vi "Main.vi"() -> ()   [LabVIEW 2022 SP3]
doc: "This sample project is built upon the standard state machine template and shows how you could create an application that acquires, analyzes, and presents data. It includes functionality for presenting configuration dialogs, preserving settings between executions, loading and saving data, as well as exporting graph images and text files.\n\nIt is most appropriate for data that is acquired instantly as it does not allow for screen updates mid acquisition nor does it allow for continuous streaming to disk."
uses:
  controls/State.ctl
  controls/Data.ctl
  controls/UI References.ctl
  controls/Graph Data.ctl
  <vilib>/Utility/miscctls.llb/LVAnnotationListTypeDef.ctl
  <vilib>/Utility/miscctls.llb/LVCursorListTypeDef.ctl
  controls/User Specified Data.ctl
  controls/HW Configuration.ctl
  controls/Analysis Configuration.ctl
  controls/New Data Behavior.ctl
panel:
  in  "Settings":bool
  in  "Snapshot":bool
  in  "Analyze":bool
  in  "Clear":bool
  in  "Exit":bool
  in  "Acquire":bool
  in  "Export":bool
  in  "Save Data":bool
  in  "Load Data":bool
  out "Graph":waveform(dbl)[](graph)
  out "Status Bar":string
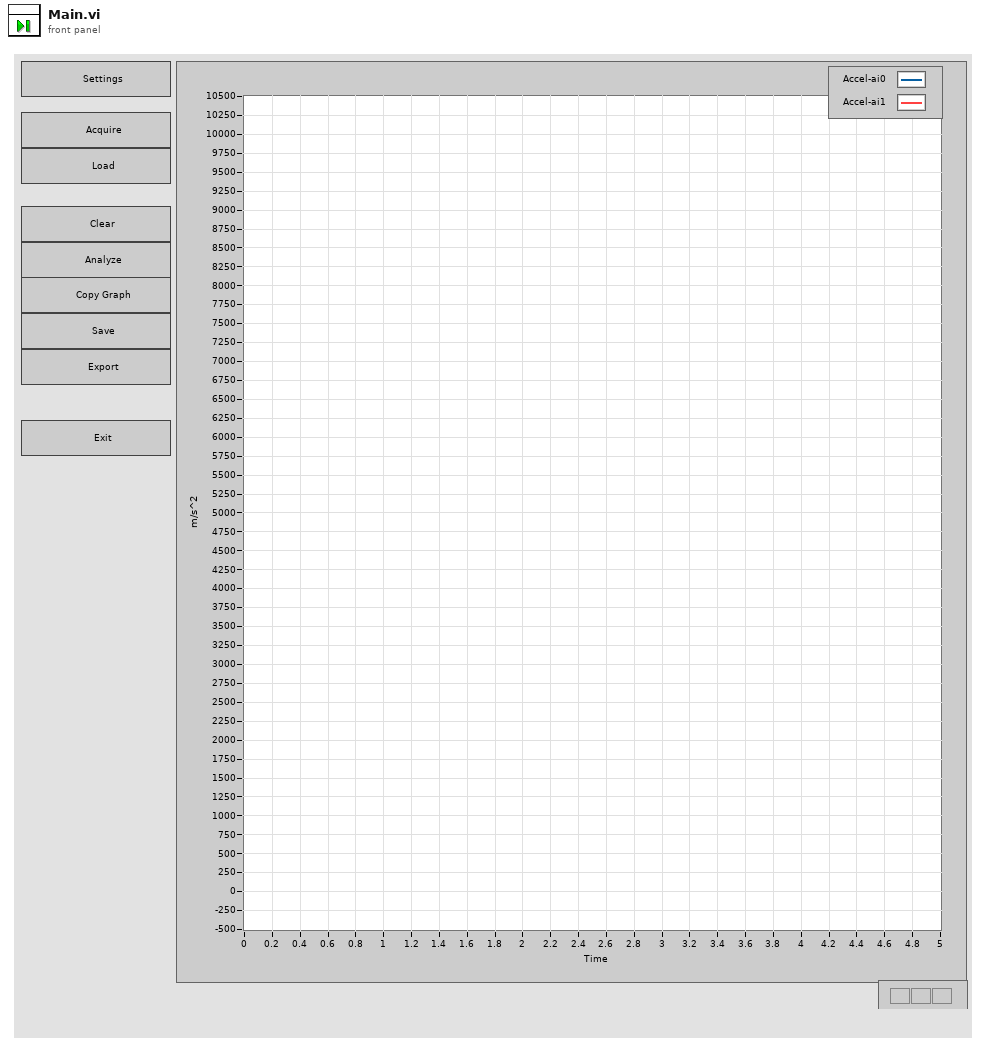
[diagram p1: front panel]
types:
  T1 = typedef "Data.ctl" = cluster{"UI References":T2, "Graph Data":T3, "User Specified":T6}
  T2 = typedef "UI References.ctl" = cluster{"Stop Ref":refnum<vi>, "Save Ref":refnum<vi>, "Open Ref":refnum<vi>, "Export Ref":refnum<vi>, "Acquire Ref":refnum<vi>, "Configure Ref":refnum<vi>, "Graph Ref":refnum<vi>, "Clear Ref":refnum<vi>, "Analyze Ref":refnum<vi>, "Status Ref":refnum<vi>, "Snapshot Ref":refnum<vi>}
  T3 = typedef "Graph Data.ctl" = cluster{"Data":waveform(dbl)[], "Annotation List":T4, "Cursor List":T5, "Analysis Data":waveform(dbl)[]}
  T4 = typedef "LVAnnotationListTypeDef.ctl" = cluster{"Name":string, "Color":u32, "Style":u8, "Point Style":u8, "Name Visible":bool, "Allow Drag":bool, "Annotation Mode":u32, "Plot":i32, "Index":i32, "Position":cluster{"X":dbl, "Y":dbl}, "X Scale":u32, "Y Scale":u32, "Show Arrow":bool, "Lock Name":bool, "Plot Area":i32, "Label Offset":cluster{"X":dbl, "Y":dbl}}[]
  T5 = typedef "LVCursorListTypeDef.ctl" = cluster{"Name":string, "Color":u32, "Style":u8, "Point Style":u8, "Name Visible":bool, "Allow Drag":bool, "Cursor Mode":u32, "Plot":i32, "Index":i32, "Position":cluster{"X":dbl, "Y":dbl}, "X Scale":u32, "Y Scale":u32, "Watch Plots":i32[], "Watch All Plots":bool, "Plot Area":i32, "Label Offset":cluster{"X":dbl, "Y":dbl}}[]
  T6 = typedef "User Specified Data.ctl" = cluster{"Hardware Configuration":T7, "Analysis Configuration":T8, "New Data Behavior":T9}
  T7 = typedef "HW Configuration.ctl" = cluster{"Accel-ai0":bool, "Maximum Input":dbl, "Minimum Input":dbl, "Sample Rate":dbl, "Number of Samples":i32, "Accel-ai1":bool}
  T8 = typedef "Analysis Configuration.ctl" = cluster{"Statistics":bool}
  T9 = typedef "New Data Behavior.ctl" = enum16{"Replace", "Overlay", "Append"}
  T10 = typedef "State.ctl" = enum16{"Initialize", "Wait for Event", "Update UI", "Configure", "Acquire", "Load Data", "Save Data", "Clear Data", "Export Data", "Analyze", "Copy Graph", "Exit"}
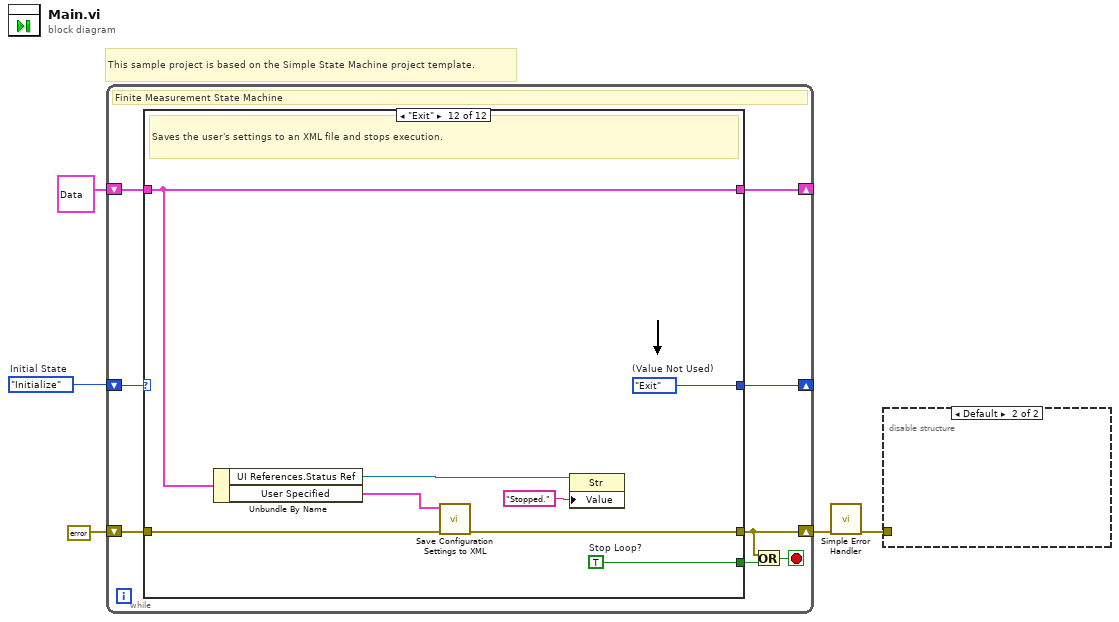
[diagram p0: block diagram]
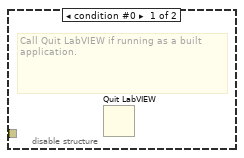
[diagram p2: hidden frame]
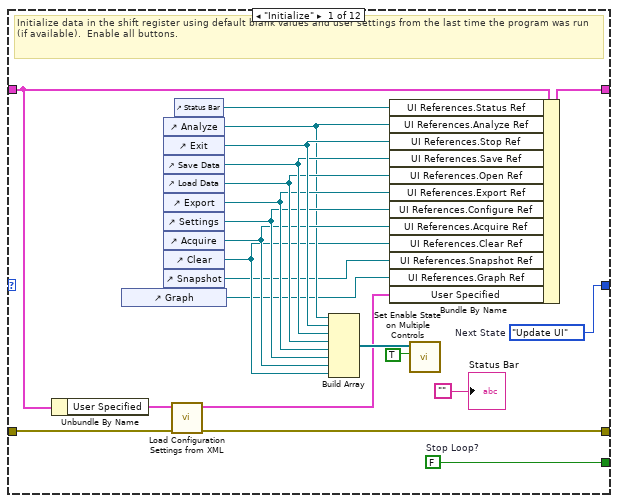
[diagram p3: hidden frame]
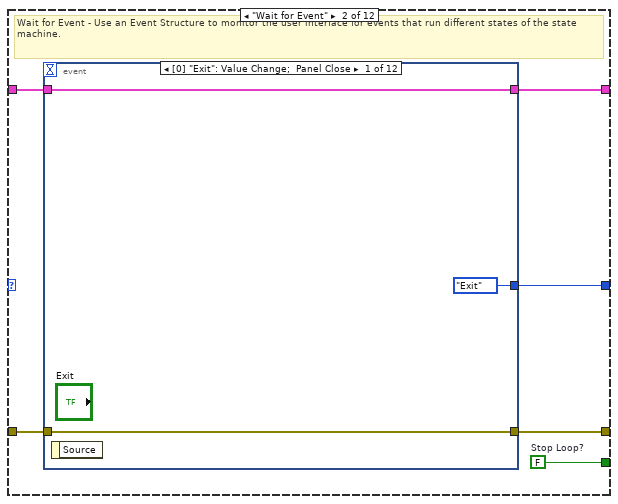
[diagram p4: hidden frame]
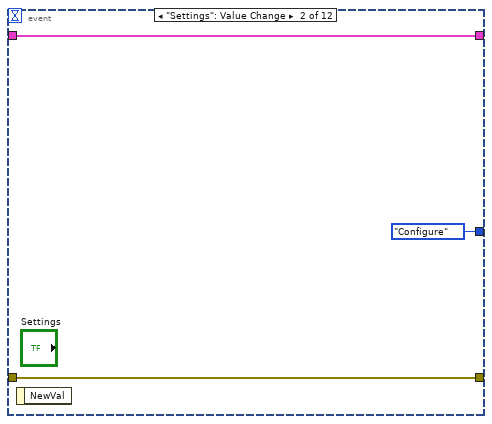
[diagram p5: hidden frame]
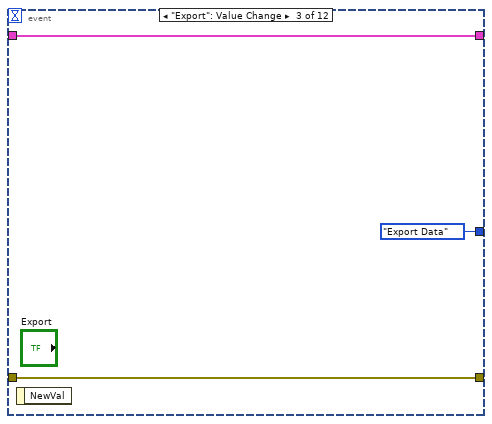
[diagram p6: hidden frame]
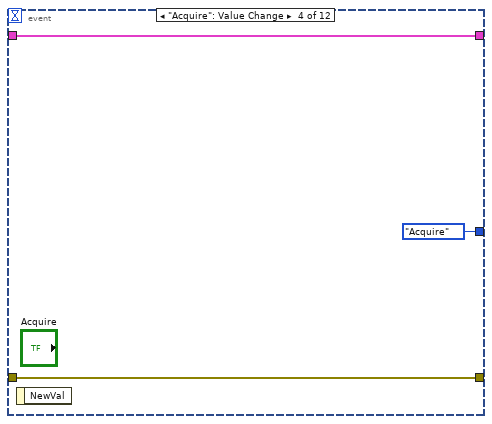
[diagram p7: hidden frame]
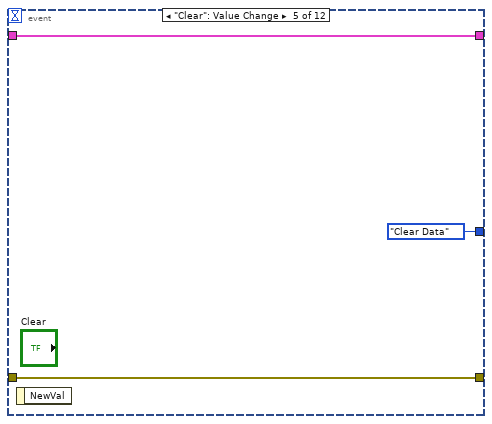
[diagram p8: hidden frame]
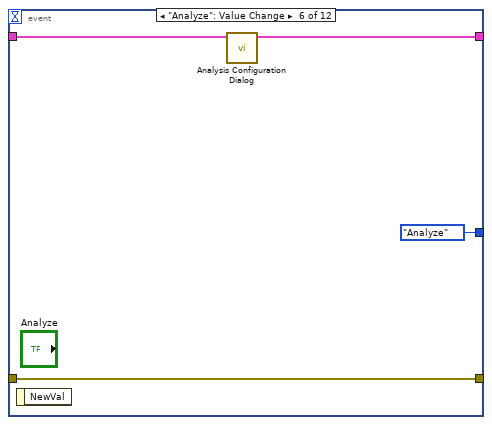
[diagram p9: hidden frame]
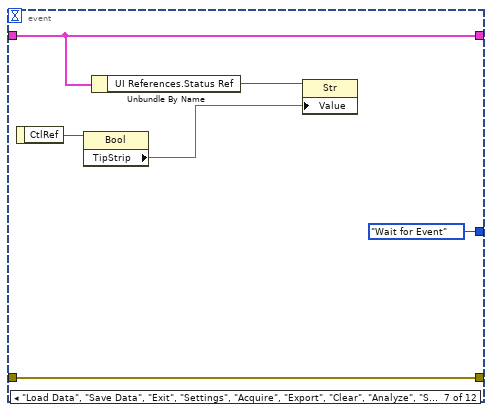
[diagram p10: hidden frame]
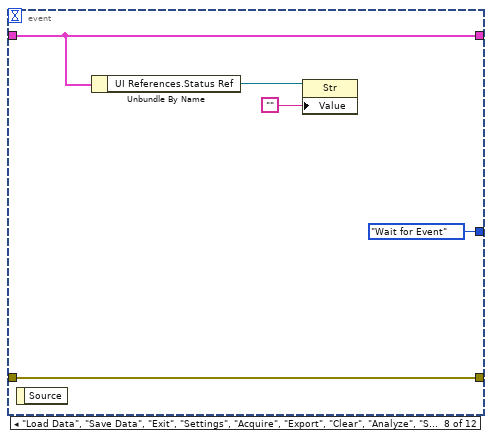
[diagram p11: hidden frame]
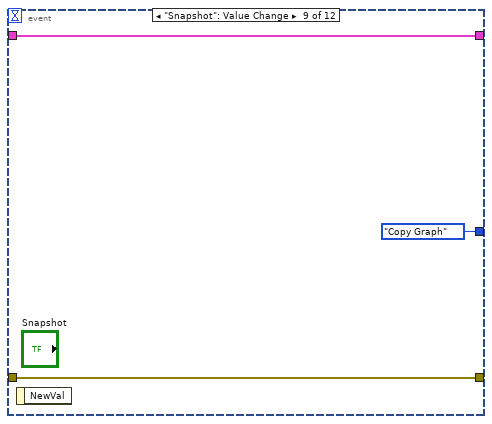
[diagram p12: hidden frame]
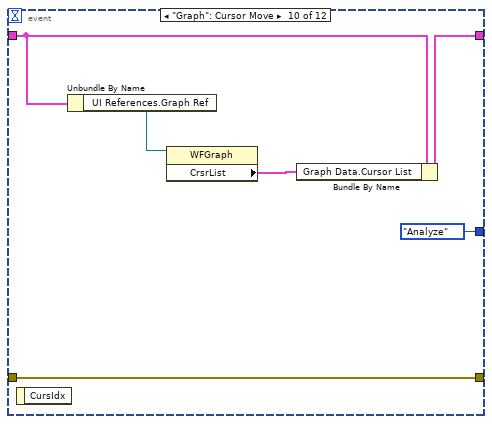
[diagram p13: hidden frame]
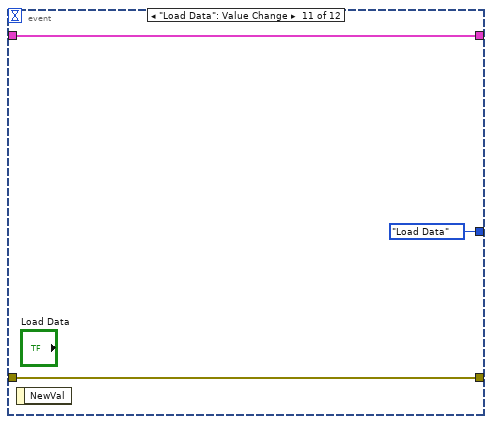
[diagram p14: hidden frame]
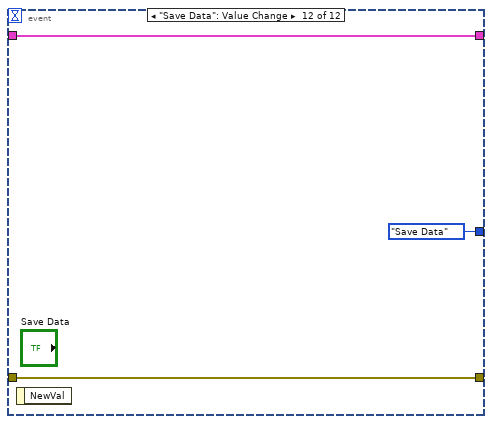
[diagram p15: hidden frame]
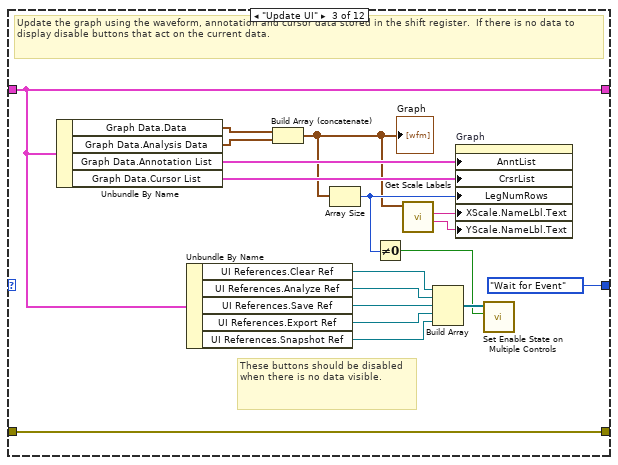
[diagram p16: hidden frame]
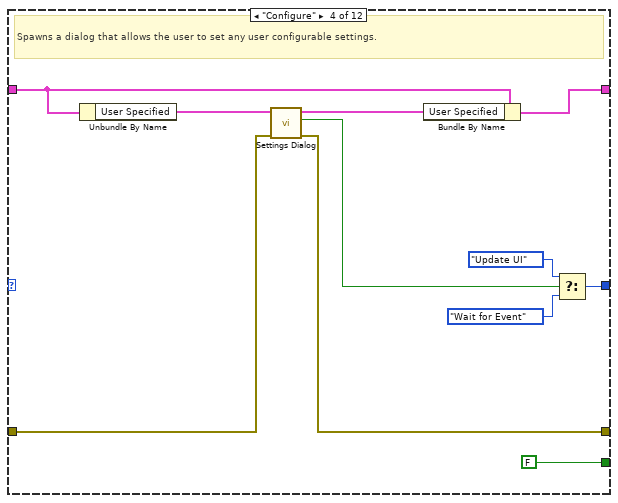
[diagram p17: hidden frame]
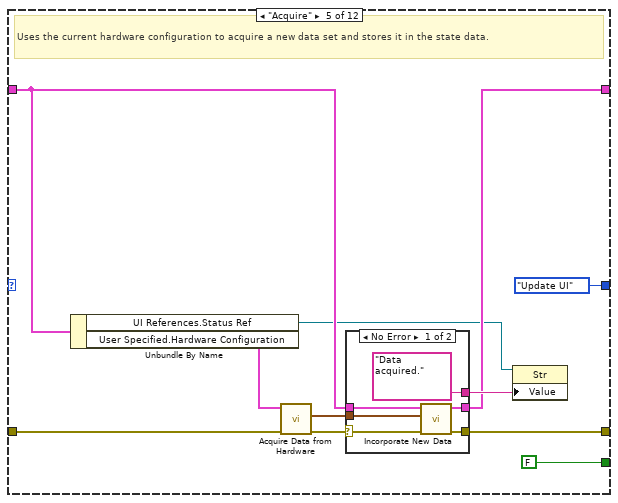
[diagram p18: hidden frame]
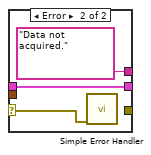
[diagram p19: hidden frame]
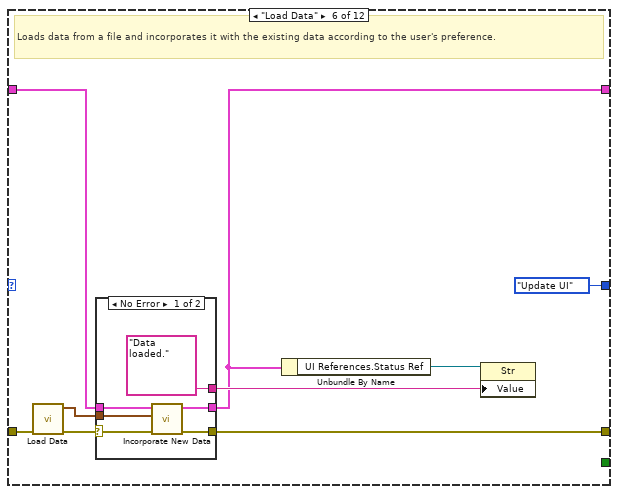
[diagram p20: hidden frame]
diagram:
  w5 = State."Initialize"  # Initial State
  # "This sample project is based on the Simple State Machine project template."
  n1 = while {
    shift-right: [w12] -> _
    shift-left: w5 -> [w13]
    shift-right: [w10] -> _
    shift-left: T1 {"UI References"={"Stop Ref"=refnum, "Save Ref"=refnum, "Open Ref"=refnum, "Export Ref"=refnum, "Acquire Ref"=refnum, "Configure Ref"=refnum, "Graph Ref"=refnum, "Clear Ref"=refnum, "Analyze Ref"=refnum, "Status Ref"=refnum, "Snapshot Ref"=refnum}, "Graph Data"={"Data"=[], "Annotation List"=[], "Cursor List"=[], "Analysis Data"=[]}, "User Specified"={"Hardware Configuration"={"Accel-ai0"=FALSE, "Maximum Input"=0.0, "Minimum Input"=0.0, "Sample Rate"=0.0, "Number of Samples"=0, "Accel-ai1"=FALSE}, "Analysis Configuration"={"Statistics"=FALSE}, "New Data Behavior"=enum."Replace"}} ("Data") -> [w11]
    shift-right: [w6] -> w2
    shift-left: errorcluster {"status"=FALSE, "code"=0, "source"=""} ("error constant") -> [w9]
    stop <- w7 stop-if-true
    # "Finite Measurement State Machine"
    n2 = case shown="\"Exit\"" w13 {
      tunnel: [w35 w41 State."Wait for Event" ("(Value Not Used)") w108 State."Update UI" ("Next State") State."Update UI" ("(Value Not Used)") State."Wait for Event" ("(Value Not Used)") State."Wait for Event" ("(Value Not Used)") State."Update UI" ("(Value Not Used)") State."Update UI" ("(Value Not Used)") State."Wait for Event" ("(Value Not Used)") w198] -> w12
      tunnel: [w34 w40 _ FALSE ("Stop Loop?") FALSE ("Stop Loop?") _ _ _ _ _ _ w197] -> w8
      tunnel: w11 -> [w25 w39 w101 w114 w121 w144 w157 w169 w180 w183 w189 w195]
      tunnel: [w33 w38 w101 w113 w120 w138 w157 w169 w179 w183 w189 w195] -> w10
      tunnel: w9 -> [w23 w37 w104 w112 w123 w143 w159 w172 w182 w185 w188 w192]
      tunnel: [w22 w36 w104 w111 w116 w142 w155 w166 w182 w185 w187 w191] -> w6
      frame "Initialize" {
        w34 = FALSE  # Stop Loop?
        w35 = State."Update UI"  # Next State
        # "Initialize data in the shift register using default blank values and user settings from the last time the program was run (if available).  Enable all buttons."
        n3 = Unbundle By Name(w25) -> ("User Specified"=w24:T6)
        n4 = control-ref of="Graph"() -> (w14:refnum<vi>)
        n5 = control-ref of="Analyze"() -> (w21:refnum<vi>)
        n6 = control-ref of="Exit"() -> (w32:refnum<vi>)
        n7 = control-ref of="Save Data"() -> (w31:refnum<vi>)
        n8 = control-ref of="Load Data"() -> (w30:refnum<vi>)
        n9 = control-ref of="Export"() -> (w29:refnum<vi>)
        n10 = control-ref of="Settings"() -> (w28:refnum<vi>)
        n11 = control-ref of="Acquire"() -> (w27:refnum<vi>)
        n12 = control-ref of="Clear"() -> (w19:refnum<vi>)
        n13 = control-ref of="Snapshot"() -> (w15:refnum<vi>)
        n14 = call "Load Configuration Settings from XML.vi"("error in (no error)"=w23, "User Configuration in"=w24) -> ("error out"=w22:errorcluster, "User Configuration out"=w17:T6)  [unwired: 8 in]
        n15 = control-ref of="Status Bar"() -> (w20:refnum<vi>)
        n16 = Build Array(w21, w32, w31, w30, w29, w28, w27, w19) -> (w26:refnum<vi>[])
        n17 = Bundle By Name(cluster=w25, "UI References.Status Ref"=w20, "UI References.Analyze Ref"=w21, "UI References.Stop Ref"=w32, "UI References.Save Ref"=w31, "UI References.Open Ref"=w30, "UI References.Export Ref"=w29, "UI References.Configure Ref"=w28, "UI References.Acquire Ref"=w27, "UI References.Clear Ref"=w19, "UI References.Snapshot Ref"=w15, "UI References.Graph Ref"=w14, "User Specified"=w17) -> (w33:T1)
        n18 = call "Set Enable State on Multiple Controls.vi"("Enable?"=TRUE, "Controls"=w26) -> ()  [unwired: 10 in]
        "Status Bar" <- "" ("Status Bar")
      }
      frame "Wait for Event" {
        w40 = FALSE  # Stop Loop?
        # "Wait for Event - Use an Event Structure to monitor the user interface for events that run different states of the state machine."
        n19 = event shown="[0] \"Exit\": Value Change;  Panel Close" {
          selector: _ -> [_ _ _ _ _ _ _ _ _ _ _ _]
          dyn-events: _ -> [_ _ _ _ _ _ _ _ _ _ _ _]
          timeout: _ -> [_ _ _ _ _ _ _ _ _ _ _ _]
          tunnel: [State."Exit" ("Next State") State."Configure" ("Next State") State."Export Data" ("Next State") State."Acquire" ("Next State") State."Clear Data" ("Next State") State."Analyze" ("Next State") State."Wait for Event" ("Next State") State."Wait for Event" ("Next State") State."Copy Graph" ("Next State") State."Analyze" ("Next State") State."Load Data" ("Next State") State."Save Data" ("Next State")] -> w41
          tunnel: w39 -> [w43 w47 w50 w53 w56 w58 w64 w70 w74 w75 w82 w85]
          tunnel: [w43 w47 w50 w53 w56 w57 w64 w70 w74 w78 w82 w85] -> w38
          tunnel: w37 -> [w42 w46 w49 w52 w55 w60 w66 w71 w73 w80 w81 w84]
          tunnel: [w42 w46 w49 w52 w55 w60 w66 w71 w73 w80 w81 w84] -> w36
          event "Exit": Value Change; Panel Close {
            n20 = event-data() -> ()  [unwired: 1 in, 1 out]
          }
          event "Settings": Value Change {
            n21 = event-data() -> ()  [unwired: 1 in, 1 out]
          }
          event "Export": Value Change {
            n22 = event-data() -> ()  [unwired: 1 in, 1 out]
          }
          event "Acquire": Value Change {
            n23 = event-data() -> ()  [unwired: 1 in, 1 out]
          }
          event "Clear": Value Change {
            n24 = event-data() -> ()  [unwired: 1 in, 1 out]
          }
          event "Analyze": Value Change {
            n25 = event-data() -> ()  [unwired: 1 in, 1 out]
            n26 = call "Analysis Configuration Dialog.vi"("Data in"=w58) -> ("Data out"=w57:T1)  [unwired: 10 in]
          }
          event "Load Data", "Save Data", "Exit", "Settings", "Acquire", "Export", "Clear", "Analyze", "Snapshot": Mouse Enter {
            n27 = event-data() -> ("CtlRef"=w65:refnum<vi>)  [unwired: 1 in]
            n28 = property class="Bool"(reference=w65) -> ("TipStrip"=w62:string)  [unwired: 1 in, 2 out]
            n29 = Unbundle By Name(w64) -> ("UI References.Status Ref"=w63:refnum<vi>)
            n30 = property class="Str"(reference=w63, "Value"=w62) -> ()  [unwired: 1 in, 2 out]
          }
          event "Load Data", "Save Data", "Exit", "Settings", "Acquire", "Export", "Clear", "Analyze", "Snapshot": Mouse Leave {
            n31 = event-data() -> ()  [unwired: 1 in, 1 out]
            n32 = Unbundle By Name(w70) -> ("UI References.Status Ref"=w69:refnum<vi>)
            n33 = property class="Str"(reference=w69, "Value"="") -> ()  [unwired: 1 in, 2 out]
          }
          event "Snapshot": Value Change {
            n34 = event-data() -> ()  [unwired: 1 in, 1 out]
          }
          event "Graph": Cursor Move {
            n35 = event-data() -> ()  [unwired: 1 in, 1 out]
            n36 = Unbundle By Name(w75) -> ("UI References.Graph Ref"=w77:refnum<vi>)
            n37 = property class="WFGraph"(reference=w77) -> ("CrsrList"=w76:T5)  [unwired: 1 in, 2 out]
            n38 = Bundle By Name(cluster=w75, "Graph Data.Cursor List"=w76) -> (w78:T1)
          }
          event "Load Data": Value Change {
            n39 = event-data() -> ()  [unwired: 1 in, 1 out]
          }
          event "Save Data": Value Change {
            n40 = event-data() -> ()  [unwired: 1 in, 1 out]
          }
        }
      }
      frame "Update UI" {
        # "These buttons should be disabled when there is no data visible."
        # "Update the graph using the waveform, annotation and cursor data stored in the shift register.  If there is no data to display disable buttons that act on the current data."
        n41 = Unbundle By Name(w101) -> ("Graph Data.Data"=w97:waveform(dbl)[], "Graph Data.Analysis Data"=w87:waveform(dbl)[], "Graph Data.Annotation List"=w102:T4, "Graph Data.Cursor List"=w98:T5)
        n42 = Unbundle By Name(w101) -> ("UI References.Clear Ref"=w93:refnum<vi>, "UI References.Analyze Ref"=w92:refnum<vi>, "UI References.Save Ref"=w100:refnum<vi>, "UI References.Export Ref"=w90:refnum<vi>, "UI References.Snapshot Ref"=w91:refnum<vi>)
        n43 = Build Array (concatenate)(w97, w87) -> (w95:waveform(dbl)[])
        "Graph" <- w95
        n44 = Array Size(array=w95) -> (size(s)=w96:i32)
        n45 = Not Equal To 0?(x=w96) -> (x != 0?=w94:bool)
        n46 = call "Get Scale Labels.vi"("Array of Waveforms"=w95) -> ("Y Scale Label Text"=w88:string, "X Scale Label Text"=w89:string)  [unwired: 9 in]
        n47 = Build Array(w93, w92, w100, w90, w91) -> (w99:refnum<vi>[])
        n48 = property on="Graph" class="WFGraph (strict)"("AnntList"=w102, "CrsrList"=w98, "LegNumRows"=w96, "XScale.NameLbl.Text"=w89, "YScale.NameLbl.Text"=w88) -> ()  [unwired: 2 in, 2 out]
        n49 = call "Set Enable State on Multiple Controls.vi"("Enable?"=w94, "Controls"=w99) -> ()  [unwired: 10 in]
      }
      frame "Configure" {
        # "Spawns a dialog that allows the user to set any user configurable settings."
        n50 = Unbundle By Name(w114) -> ("User Specified"=w106:T6)
        n51 = call "Settings Dialog.vi"("error in (no error)"=w112, "Configuration in"=w106) -> ("error out"=w111:errorcluster, "UI Refresh Needed?"=w110:bool, "Configuration out"=w105:T6)  [unwired: 7 in]
        n52 = Bundle By Name(cluster=w114, "User Specified"=w105) -> (w113:T1)
        n53 = Select(t=State."Update UI" ("Next State if true"), s=w110, f=State."Wait for Event" ("Next State if false")) -> (s? t:f=w108:T10)
      }
      frame "Acquire" {
        # "Uses the current hardware configuration to acquire a new data set and stores it in the state data."
        n54 = Unbundle By Name(w121) -> ("UI References.Status Ref"=w117:refnum<vi>, "User Specified.Hardware Configuration"=w124:T7)
        n55 = call "Acquire Data from Hardware.vi"("error in (no error)"=w123, "Hardware Configuration"=w124) -> ("error out"=w118:errorcluster, "Graph Data"=w119:waveform(dbl)[])  [unwired: 7 in]
        n56 = case shown="No Error" w118 {
          selector: w118 -> [w129 w134]
          tunnel: w121 -> [w128 w135]
          tunnel: [w132 w135] -> w120
          tunnel: [w131 _] -> w116
          tunnel: w119 -> [w130 _]
          tunnel: ["Data acquired." ("Data acquired") "Data not acquired." ("Data not acquired")] -> w122
          frame No Error {
            n57 = call "Incorporate New Data.vi"("error in (no error)"=w129, "New Graph Data"=w130, "Data in"=w128) -> ("error out"=w131:errorcluster, "Data out"=w132:T1)  [unwired: 7 in]
          }
          frame Error {
            n58 = call <vilib>:"Simple Error Handler.vi"("error in (no error)"=w134) -> ()  [unwired: 4 in, 5 out]
          }
        }
        n59 = property class="Str"(reference=w117, "Value"=w122) -> ()  [unwired: 1 in, 2 out]
      }
      frame "Load Data" {
        # "Loads data from a file and incorporates it with the existing data according to the user's preference."
        n60 = call "Load Data.vi"("error in (no error)"=w143) -> ("error out"=w140:errorcluster, "New Graph Data"=w137:waveform(dbl)[])  [unwired: 9 in]
        n61 = case shown="No Error" w140 {
          selector: w140 -> [w147 w152]
          tunnel: w144 -> [w146 w153]
          tunnel: [w150 w153] -> w138
          tunnel: [w149 _] -> w142
          tunnel: w137 -> [w148 _]
          tunnel: ["Data loaded." ("Data loaded") "Data not loaded." ("Data not loaded")] -> w139
          frame No Error {
            n62 = call "Incorporate New Data.vi"("error in (no error)"=w147, "New Graph Data"=w148, "Data in"=w146) -> ("error out"=w149:errorcluster, "Data out"=w150:T1)  [unwired: 7 in]
          }
          frame Error {
            n63 = call <vilib>:"Simple Error Handler.vi"("error in (no error)"=w152) -> ()  [unwired: 4 in, 5 out]
          }
        }
        n64 = Unbundle By Name(w138) -> ("UI References.Status Ref"=w136:refnum<vi>)
        n65 = property class="Str"(reference=w136, "Value"=w139) -> ()  [unwired: 1 in, 2 out]
      }
      frame "Save Data" {
        # "Saves the existing measurement data to a file."
        n66 = Unbundle By Name(w157) -> ("UI References.Status Ref"=w156:refnum<vi>, "Graph Data.Data"=w160:waveform(dbl)[])
        n67 = call "Save Data.vi"("error in (no error)"=w159, "Data"=w160) -> ("error out"=w158:errorcluster)  [unwired: 9 in]
        n68 = case shown="No Error" w158 {
          selector: w158 -> [w162 w165]
          tunnel: ["Data saved." ("Data saved") "Data not saved." ("Data not saved")] -> w154
          tunnel: [w162 _] -> w155
          frame No Error {
          }
          frame Error {
            n69 = call <vilib>:"Simple Error Handler.vi"("error in (no error)"=w165) -> ()  [unwired: 4 in, 5 out]
          }
        }
        n70 = property class="Str"(reference=w156, "Value"=w154) -> ()  [unwired: 1 in, 2 out]
      }
      frame "Export Data" {
        # "Exports the currently loaded measurement and analysis data to a text file that can be imported into a spreadsheet or other application."
        n71 = Unbundle By Name(w169) -> ("UI References.Status Ref"=w167:refnum<vi>, "Graph Data"=w168:T3)
        n72 = call "Export Data.vi"("error in (no error)"=w172, "Graph Data"=w168) -> ("error out"=w170:errorcluster)  [unwired: 9 in]
        n73 = case shown="No Error" w170 {
          selector: w170 -> [w174 w177]
          tunnel: ["Data exported." ("Data exported") "Data not exported." ("Data not exported")] -> w171
          tunnel: [w174 _] -> w166
          frame No Error {
          }
          frame Error {
            n74 = call <vilib>:"Simple Error Handler.vi"("error in (no error)"=w177) -> ()  [unwired: 4 in, 5 out]
          }
        }
        n75 = property class="Str"(reference=w167, "Value"=w171) -> ()  [unwired: 1 in, 2 out]
      }
      frame "Clear Data" {
        # "Clears the data currently in the graph."
        n76 = Bundle By Name(cluster=w180, "Graph Data"=T3 {"Data"=[], "Annotation List"=[], "Cursor List"=[], "Analysis Data"=[]} ("Graph")) -> (w179:T1)
      }
      frame "Analyze" {
        # "#CodeRecommended - add your own signal analysis here."
        # "Analyzes the measurement data using the user selected routines and adds annotations and calculated channels to the graph where appropriate."
        n77 = Unbundle By Name(w183) -> ("Graph Data"=w184:T3)
        n78 = call "Statistical Analysis.vi"("Graph Data In"=w184) -> ()  [unwired: 8 in, 2 out]
      }
      frame "Copy Graph" {
        # "Places an image of the graph on the clipboard for pasting into reports or emails."
        n79 = call "Copy Graph to Clipboard.vi"("error in (no error)"=w188, "Graph Data"=w189) -> ("error out"=w187:errorcluster)  [unwired: 9 in]
      }
      frame "Exit" {
        w197 = TRUE  # Stop Loop?
        w198 = State."Exit"  # (Value Not Used)
        # "Saves the user's settings to an XML file and stops execution."
        n80 = Unbundle By Name(w195) -> ("UI References.Status Ref"=w193:refnum<vi>, "User Specified"=w196:T6)
        n81 = call "Save Configuration Settings to XML.vi"("error in (no error)"=w192, "User Configuration"=w196) -> ("error out"=w191:errorcluster)  [unwired: 9 in]
        n82 = property class="Str"(reference=w193, "Value"="Stopped." ("Stopped")) -> ()  [unwired: 1 in, 2 out]
      }
    }
    n83 = Or(x=w6, y=w8) -> (x .or. y?=w7:bool)
  }
  n84 = call <vilib>:"Simple Error Handler.vi"("error in (no error)"=w2) -> ("error out"=w1:errorcluster)  [unwired: 4 in, 4 out]
  n85 = disable-structure shown="Default" {
    disable-tunnel: w1 -> [_ _]
    frame condition #0 {
      # "Call Quit LabVIEW if running as a built application."
      n86 = Quit LabVIEW() -> ()  [unwired: 1 in]
    }
    frame condition #1 (active) {
    }
  }
